vi "origin.vi"(10 "zorg":dbl, 11 "xorg":dbl) -> ()   [LabVIEW 2017, in "HapticSTM.lvlib"]
doc: "extern \"C\" __declspec(dllexport) void origin(double xorg, double zorg);"
uses:
  <userlib>/HapticSTM/Feedbackless - Testdata/Project/HapticSTM.lvlib
  <userlib>/HapticSTM/HapticSTM.dll
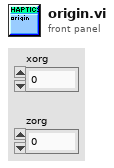
[diagram p1: front panel]
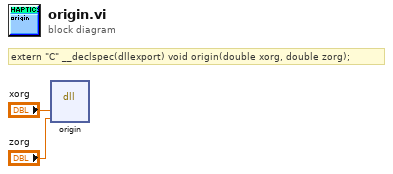
[diagram p0: block diagram]
diagram:
  # "extern \"C\" __declspec(dllexport) void origin(double xorg, double zorg);"
  n1 = dll-call lib="C:/Program Files/National Instruments/LabVIEW 2019/user.lib/HapticSTM/HapticSTM.*" fn="origin"("xorg"="xorg", "zorg"="zorg") -> ()  [unwired: 6 in, 2 out]
